vi "MCB2400 AO PrjAttrValidator.vi"(5 "Ctl Refnum":refnum<vi>, 9 "Numeric":u8, 11 "Attributes":T1 {"Programmable Pin Connections" items=["AOUT0 uses pin P0.26 (also used by AI3). You cannot use AOUT0 and pin P0.26 (or AI3) in the same project."]}) -> (3 "Valid?":bool)   [LabVIEW 2011]
uses:
  <vilib>/Embedded/ARM/MCB2400/MCB2400_AO_PrjAttr.ctl
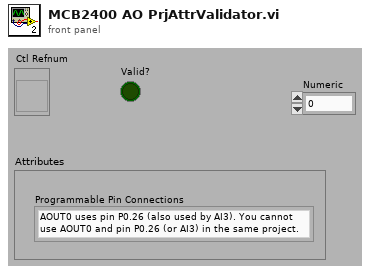
[diagram p1: front panel]
types:
  T1 = typedef "MCB2400_AO_PrjAttr.ctl" = cluster{"Programmable Pin Connections":u16}
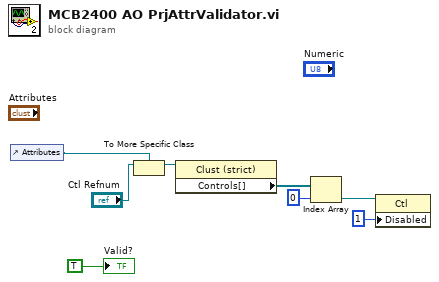
[diagram p0: block diagram]
diagram:
  n1 = control-ref of="Attributes"() -> (w1:refnum<vi>)
  n2 = To More Specific Class(target class=w1, reference="Ctl Refnum") -> (specific class reference=w3:refnum<vi>)  [unwired: 1 in, 1 out]
  n3 = property class="Clust (strict)"(reference=w3) -> ("Controls[]"=w7:refnum<vi>[])  [unwired: 1 in, 2 out]
  n4 = Index Array(array=w7, index=0) -> (element=w5:refnum<vi>)
  n5 = property class="Ctl"(reference=w5, "Disabled"=u8 1) -> ()  [unwired: 1 in, 2 out]
  "Valid?" <- TRUE ("Valid?")
